vi "String to 1D I64 Array.vi"(4 "Delimiter (,)":string=",", 6 "String":string) -> (1 "Array[]":i64[](array[numeric]))   [LabVIEW 2016, in "SLL String.lvlib"]
uses:
  SLL String.lvlib
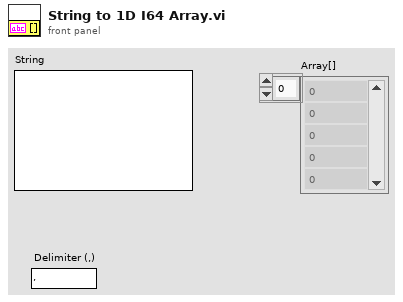
[diagram p1: front panel]
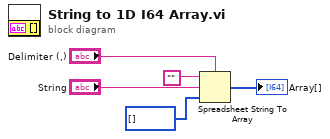
[diagram p0: block diagram]
diagram:
  n1 = Spreadsheet String To Array(delimiter (Tab)="Delimiter (,)", format string="", spreadsheet string="String", array type (2D Dbl)=i64[] []) -> (array=→"Array[]":i64[])
